vi "Set Sparse Points.vi"(4 "Side":T1=enum."right") -> ()   [LabVIEW 2013]
uses:
  ROS/Code/SubVIs/BaxterSide.ctl
  Baxter Examples/Arm Globals.vi
  <vilib>/Utility/config.llb/Read Key (Double).vi
  Prim/Fwd Kenimatics - array.vi
  <vilib>/Utility/config.llb/NI_LVConfig.lvlib
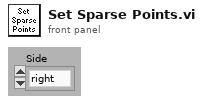
[diagram p1: front panel]
types:
  T1 = typedef "BaxterSide.ctl" = enum16{"left", "right"}
  T2 = cluster{"J[0]":dbl, "J[1]":dbl, "J[2]":dbl, "J[3]":dbl, "J[4]":dbl, "J[5]":dbl, "J[6]":dbl}
  T3 = cluster{"Label":string, "Joints":dbl[], "Far Left":cluster{"Absolute":dbl[], "Robot":dbl[]}, "Far Right":cluster{"Absolute":dbl[], "Robot":dbl[]}, "Near Left":cluster{"Absolute":dbl[], "Robot":dbl[]}, "Near Right":cluster{"Absolute":dbl[], "Robot":dbl[]}}[]
  T4 = typedef "NI_Matrix.lvlib/RealMatrix.ctl" = dbl[][]
  T5 = cluster{"Label":string, "Joints":dbl[], "T":T4}[]
  T6 = typedef "NI_LVConfig.lvlib/Config Data RefNum.ctl" = refnum<k1>
  T7 = cluster{"J[0]":dbl, "J[1]":dbl, "J[2]":dbl, "J[3]":dbl, "J[4]":dbl, "J[5]":dbl, "J[6]":dbl}[]
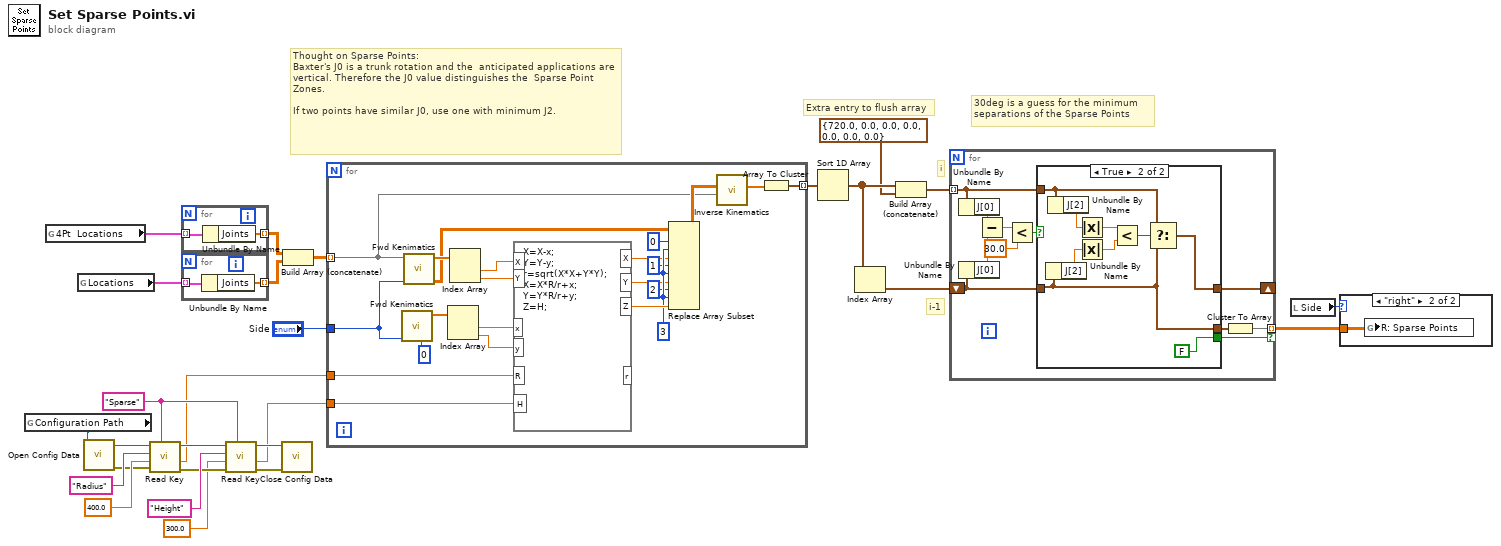
[diagram p0: block diagram]
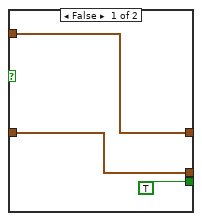
[diagram p2: hidden frame]
diagram:
  w23 = "Sparse"
  # "30deg is a guess for the minimum\nseparations of the Sparse Points"
  # "Extra entry to flush array"
  # "i-1"
  # "i"
  # "Thought on Sparse Points:\nBaxter's J0 is a trunk rotation and the  anticipated applications are vertical. Therefore the J0 value distinguishes the  Sparse Point Zones.\n\nIf two points have similar J0, use one with minimum J2."
  n1 = global read "Arm Globals.vi" "Configuration Path"() -> (w27:path)
  n2 = global read "Arm Globals.vi" "4Pt  Locations"() -> (w13:T3)
  n3 = global read "Arm Globals.vi" "Locations"() -> (w12:T5)
  n4 = call <vilib>:"Open Config Data.vi"("configuration file path"=w27) -> ("error out"=w20:errorcluster, "refnum"=w26:T6)  [unwired: 8 in, 1 out]
  n5 = call-poly <vilib>:"Read Key.vi"("section"=w23, "error in (no error)"=w20, "default value"=400.0, "key"="Radius", "refnum"=w26) -> ("error out"=w19:errorcluster, "value"=w15:dbl, "refnum out"=w24:T6)  [unwired: 3 in, 1 out]
  n6 = for {
    tunnel: w13 -> [w29] mode=indexing
    tunnel: [w28] -> w11 mode=indexing
    n7 = Unbundle By Name(w29) -> ("Joints"=w28:dbl[])
  }
  n8 = for {
    tunnel: w12 -> [w31] mode=indexing
    tunnel: [w30] -> w10 mode=indexing
    n9 = Unbundle By Name(w31) -> ("Joints"=w30:dbl[])
  }
  n10 = call-poly <vilib>:"Read Key.vi"("section"=w23, "error in (no error)"=w19, "default value"=300.0, "key"="Height", "refnum"=w24) -> ("error out"=w16:errorcluster, "value"=w14:dbl, "refnum out"=w17:T6)  [unwired: 3 in, 1 out]
  n11 = call <vilib>:"Close Config Data.vi"("error in (no error)"=w16, "refnum"=w17) -> ()  [unwired: 8 in, 2 out]
  n12 = Build Array (concatenate)(w11, w10) -> (w9:dbl[][])
  n13 = for {
    tunnel: w15 -> [w49]
    tunnel: w14 -> [w45]
    tunnel: w9 -> [w37] mode=indexing
    tunnel: "Side" -> [w34]
    tunnel: [w32] -> w6 mode=indexing
    w41 = 3 ("disabled index (col)")
    n14 = call-poly "Fwd Kenimatics.vi"("To"=0, "Side"=w34) -> ("Position"=w48:dbl[])  [unwired: 8 in, 1 out]
    n15 = call-poly "Fwd Kenimatics.vi"("Side"=w34, "Joints"=w37) -> ("Matrix"=w44:T4, "Position"=w52:dbl[])  [unwired: 8 in]
    n16 = Index Array(array=w48) -> (element #1=w46:dbl, element #2=w47:dbl)  [unwired: 2 in]
    n17 = Index Array(array=w52) -> (element #1=w51:dbl, element #2=w50:dbl)  [unwired: 2 in]
    n18 = formula code="X=X-x;\nY=Y-y;\nr=sqrt(X*X+Y*Y);\nX=X*R/r+x;\nY=Y*R/r+y;\nZ=H;"("R"=w49, "X"=w51, "Y"=w50, "x"=w46, "y"=w47, "H"=w45) -> ("X"=w36:dbl, "Y"=w35:dbl, "Z"=w43:dbl)  [unwired: 1 out]
    n19 = Replace Array Subset(array=w44, new element #1=w36, index (row) #1=0 ("disabled index (row)"), index (col) #1=w41, new element #2=w35, index (row) #2=1 ("disabled index (row)"), index (col) #2=w41, new element #3=w43, index (row) #3=2 ("disabled index (row)"), index (col) #3=w41) -> (w38:T4)
    n20 = call "Inverse Kinematics.vi"("Start"=w37, "Goal-matrix"=w38) -> ("J"=w33:dbl[])  [unwired: 6 in, 3 out]
    n21 = Array To Cluster(array=w33) -> (cluster=w32:T2)
  }
  n22 = Sort 1D Array(array=w6) -> (sorted array=w3:T7)
  n23 = Index Array(array=w3) -> (element=w4:T2)  [unwired: 1 in]
  n24 = Build Array (concatenate)(w3, T2 {"J[0]"=720.0, "J[1]"=0.0, "J[2]"=0.0, "J[3]"=0.0, "J[4]"=0.0, "J[5]"=0.0, "J[6]"=0.0} ("cluster")) -> (w1:T7)
  n25 = for {
    tunnel: w1 -> [w58] mode=indexing
    tunnel: [w64] -> w5 mode=indexing if=w55
    shift-right: [w54] -> _
    shift-left: w4 -> [w57]
    n26 = Unbundle By Name(w58) -> ("J[0]"=w61:dbl)
    n27 = Unbundle By Name(w57) -> ("J[0]"=w60:dbl)
    n28 = Subtract(x=w61, y=w60) -> (x-y=w63:dbl)
    n29 = Less?(x=w63, y=30.0) -> (x < y?=w59:bool)
    n30 = case shown="True" w59 {
      tunnel: w58 -> [w65 w70]
      tunnel: w57 -> [w67 w69]
      tunnel: [w67 w69] -> w56
      tunnel: [TRUE FALSE] -> w55
      tunnel: [w65 w68] -> w54
      frame False {
      }
      frame True {
        n31 = Unbundle By Name(w69) -> ("J[2]"=w74:dbl)
        n32 = Unbundle By Name(w70) -> ("J[2]"=w75:dbl)
        n33 = Absolute Value(x=w75) -> (abs(x)=w73:dbl)
        n34 = Absolute Value(x=w74) -> (abs(x)=w72:dbl)
        n35 = Less?(x=w73, y=w72) -> (x < y?=w71:bool)
        n36 = Select(t=w70, s=w71, f=w69) -> (s? t:f=w68:T2)
      }
    }
    n37 = Cluster To Array(cluster=w56) -> (array=w64:dbl[])
  }
  n38 = local read "Side"() -> (w7:T1)
  n39 = case shown="\"right\"" w7 {
    tunnel: w5 -> [_ w77]
    frame "left", Default {
    }
    frame "right" {
      n40 = global write "Arm Globals.vi" "R: Sparse Points"(w77) -> ()
    }
  }
